vi "simple_continous_read.vi"() -> ()   [LabVIEW 2013]
doc: "This example illustrate how to use some of the VI included in the OpenBCI toolbox"
uses:
  Comm Protocol/Control Def/channel_count.ctl
panel:
  out "CH1":dbl[](graph)
  in  "channel_count(8)":T1
  out "sample count":dbl[](graph)
  in  "stop":bool
  out "EEG Waveform Channels 1 - 8":dbl[][](graph)
  out "Console":string
  in  "COM port":refnum<visa-resource-name>
  # "Instructions:\nBefore running the VI\n1. Select the COM port for the OpenBCI receiver\n2. Select the number of channels in your board\n3. Run the VI\n4. The Device initial response is shown in the Console textbox  \n5. Click on \"Stop\" to stop the EEG acquisition"
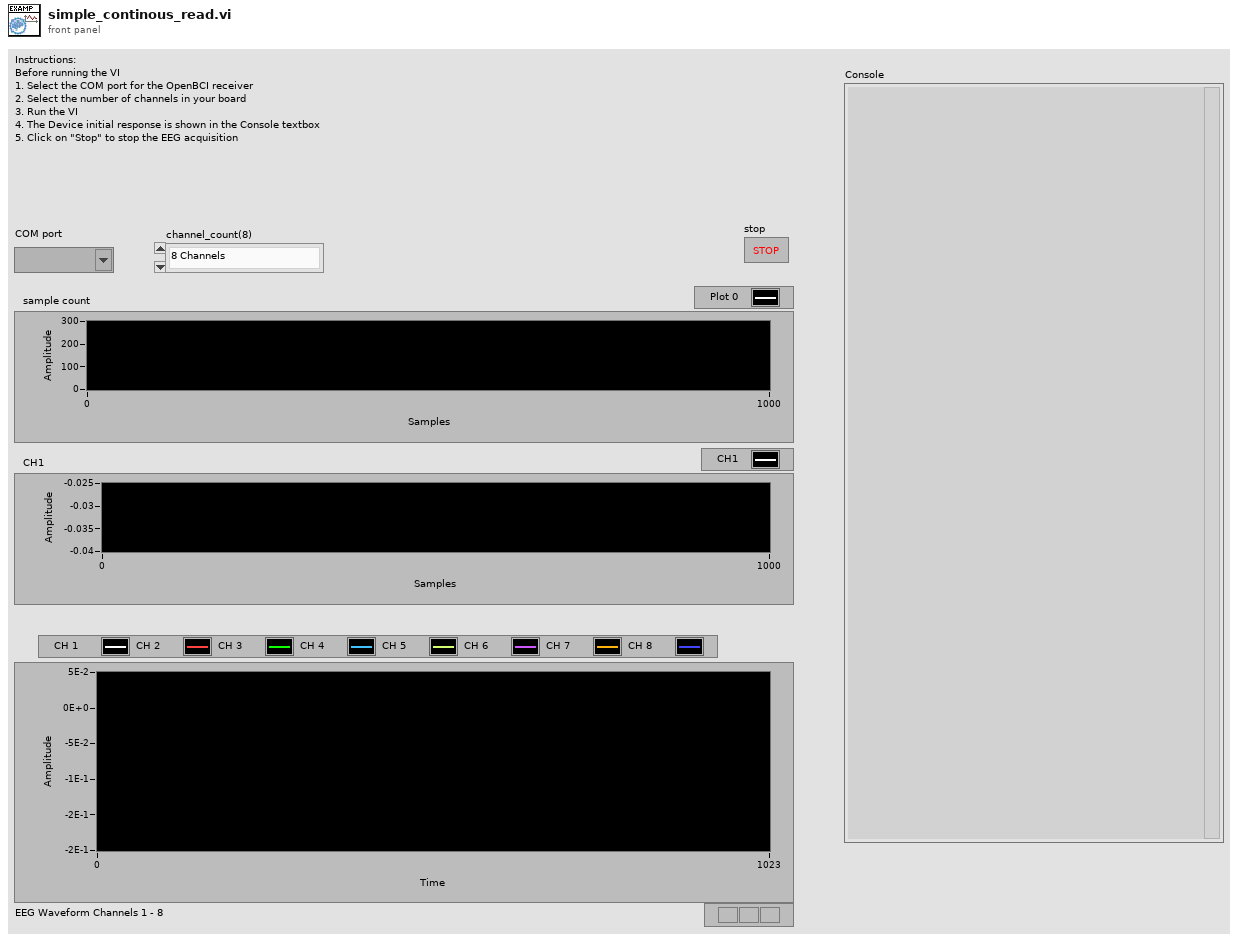
[diagram p1: front panel]
types:
  T1 = typedef "channel_count.ctl" = enum16{"8 Channels", "16 Channels"}
  T2 = typedef "openbci_device.ctl" = cluster{"COM port":refnum<visa-resource-name>, "n_ch (8)":T1, "delay_tx":u32}
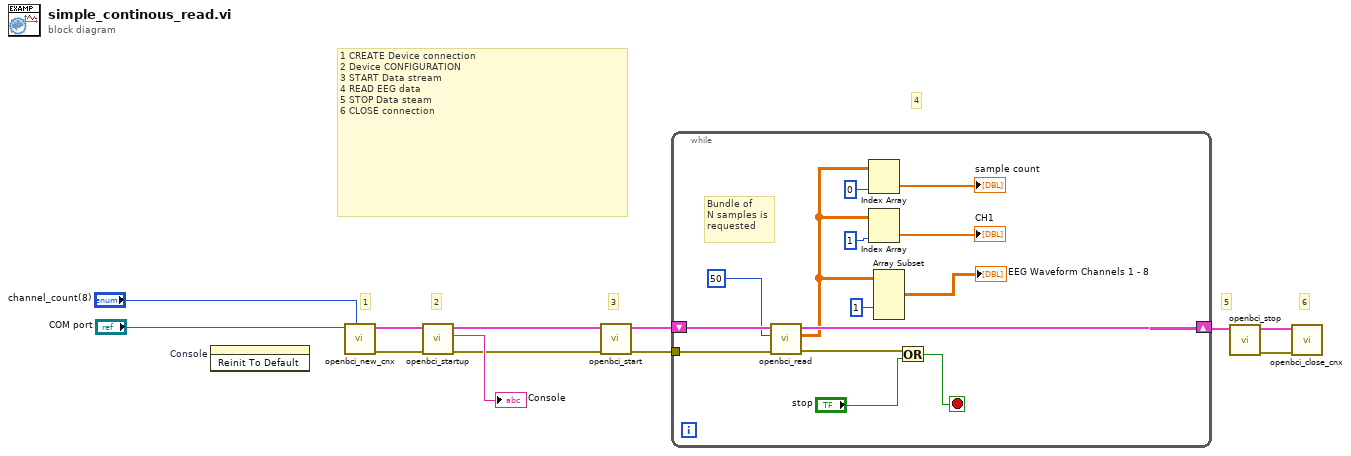
[diagram p0: block diagram]
diagram:
  # "1"
  # "4"
  # "6"
  # "5"
  # "3"
  # "2"
  # "1 CREATE Device connection\n2 Device CONFIGURATION\n3 START Data stream \n4 READ EEG data\n5 STOP Data steam\n6 CLOSE connection"
  n1 = invoke on="Console" class="Str" method="Reinit To Default"() -> ()  [unwired: 3 in, 3 out]
  n2 = call "openbci_new_cnx.vi"("channel_count(8)"="channel_count(8)", "COM port"="COM port") -> ("error out"=w7:errorcluster, "OBCI dev out"=w4:T2)  [unwired: 8 in]
  n3 = call "openbci_startup.vi"("error in"=w7, "OBCI dev in"=w4) -> ("error out"=w8:errorcluster, "start_up_string"=→"Console":string, "OBCI dev out"=w3:T2)  [unwired: 7 in]
  n4 = call "openbci_start.vi"("error in (no error)"=w8, "OBCI dev in"=w3) -> ("error out"=w9:errorcluster, "OBCI dev out"=w10:T2)  [unwired: 8 in]
  n5 = while {
    shift-right: [w25] -> w11
    shift-left: w10 -> [w26]
    tunnel: w9 -> [w23]
    stop <- w21 stop-if-true
    # "Bundle of \nN samples is\nrequested"
    n6 = call "openbci_read.vi"("error in"=w23, "N samples (2)"=50, "OBCI dev in"=w26) -> ("error out"=w22:errorcluster, "EEG data"=w13:dbl[][], "OBCI dev out"=w25:T2)  [unwired: 5 in, 1 out]
    n7 = Index Array(array=w13, index (col)=0 ("disabled index (col)")) -> (element=→"sample count":dbl[])  [unwired: 1 in]
    n8 = Index Array(array=w13, index (col)=1 ("disabled index (col)")) -> (element=→"CH1":dbl[])  [unwired: 1 in]
    n9 = Array Subset(array=w13, index (col)=1 ("index")) -> (→"EEG Waveform Channels 1 - 8":dbl[][])  [unwired: 3 in]
    n10 = Or(x=w22, y="stop") -> (x .or. y?=w21:bool)
  }
  n11 = call "openbci_stop.vi"("OBCI dev in"=w11) -> ("error out"=w1:errorcluster, "OBCI dev out"=w2:T2)  [unwired: 9 in]
  n12 = call "openbci_close_cnx.vi"("error in (no error)"=w1, "OBCI dev in"=w2) -> ()  [unwired: 9 in, 1 out]
